vi "UIEnable.vi"(0 "CmdLib In":refnum<k24>, 5 "Status:":refnum<vi>, 7 "UI":T1, 9 "Device Array":T2(array[cluster]), 11 "error in":errorcluster) -> (15 "error out":errorcluster)   [LabVIEW 2020]
uses:
  C:/GEECS/Developers Version/source/Device Drivers/Picomotor8742dotNet/NewFocus/CmdLib.dll
  NewFocus/CmdLib.dll
  Global Variables.vi
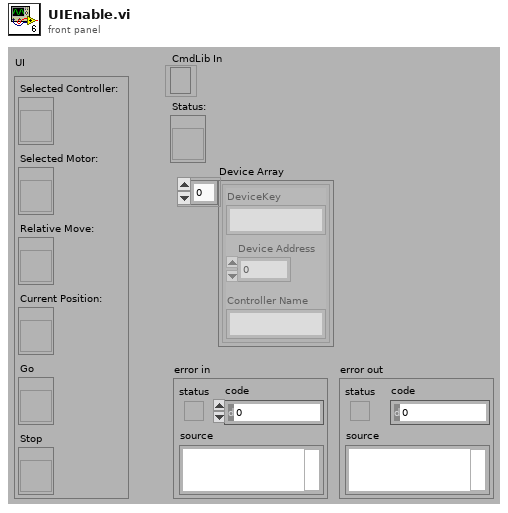
[diagram p1: front panel]
types:
  T1 = cluster{"Selected Controller:":refnum<vi>, "Selected Motor:":refnum<vi>, "Relative Move:":refnum<vi>, "Current Position:":refnum<vi>, "Go":refnum<vi>, "Stop":refnum<vi>}
  T2 = cluster{"DeviceKey":string, "Device Address":i32, "Controller Name":string}[]
  T3 = enum8{"Enabled", "Disabled", "Disabled and Grayed Out"}
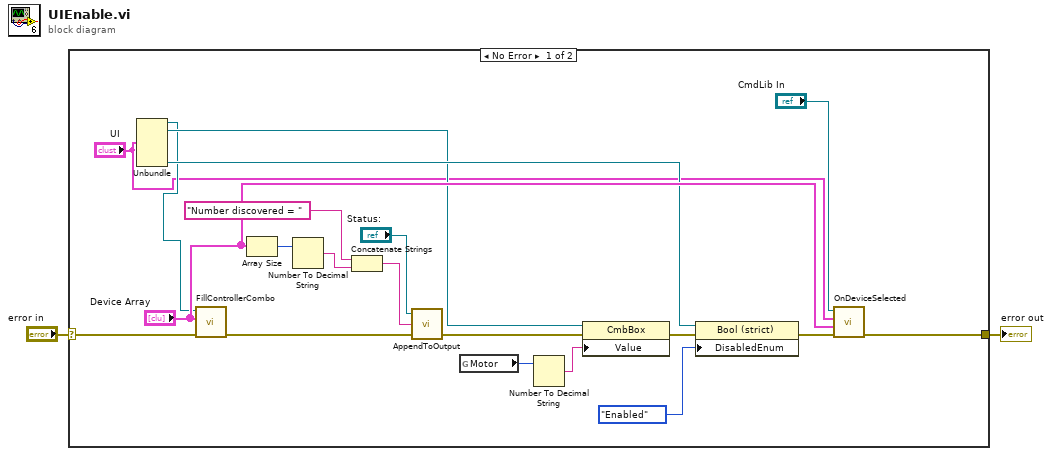
[diagram p0: block diagram]
diagram:
  n1 = case shown="No Error" "error in" {
    selector: "error in" -> [w16 w23]
    tunnel: [w18 w23] -> w2
    frame No Error {
      n2 = Unbundle("UI") -> ("Selected Controller:"=w4:refnum<vi>, "Selected Motor:"=w5:refnum<vi>, "Stop"=w6:refnum<vi>)  [unwired: 3 out]
      n3 = call "FillControllerCombo.vi"("error in (no error)"=w16, "Device Array"="Device Array", "Selected Controller:"=w4) -> ("error out"=w15:errorcluster)  [unwired: 8 in]
      n4 = Array Size(array="Device Array") -> (size(s)=w17:i32)
      n5 = Number To Decimal String(number=w17) -> (decimal integer string=w20:string)  [unwired: 1 in]
      n6 = Concatenate Strings("Number discovered = " ("string"), w20) -> (w22:string)
      n7 = call "AppendToOutput.vi"("error in"=w15, "Input String"=w22, "Output Refnum In"="Status:") -> ("error out"=w10:errorcluster)  [unwired: 1 in, 1 out]
      n8 = global read "Global Variables.vi" "Motor"() -> (w13:i32)
      n9 = Number To Decimal String(number=w13) -> (decimal integer string=w14:string)  [unwired: 1 in]
      n10 = property class="CmbBox"(reference=w5, error in=w10, "Value"=w14) -> (error out=w8:errorcluster)  [unwired: 1 out]
      n11 = property class="Bool (strict)"(reference=w6, error in=w8, "DisabledEnum"=T3."Enabled" ("Disabled")) -> (error out=w7:errorcluster)  [unwired: 1 out]
      n12 = call "OnDeviceSelected.vi"("error in"=w7, "Device Array"="Device Array", "UI"="UI", "CmdLib In"="CmdLib In") -> ("error out"=w18:errorcluster)  [unwired: 7 in]
    }
    frame Error {
    }
  }
  "error out" <- w2
